vi "FTW-Request-Unknown.vi"(0 "Request":refnum<data-value>, 11 "error in":errorcluster) -> (4 "Request out":refnum<data-value>, 15 "error out":errorcluster)   [LabVIEW 2015]
uses:
  json/core/FTW-JSON-Core-Structure.ctl
  error/FTW-ERR-ThrowError.vi
  error/FTW-ERR-CallChain.vi
  error/FTW-ERR-NoErrorConstant.vi
  string/FTW-STR-ReplaceWhitespace.vi
  string/FTW-STR-Array-Delimit.vi
  error/FTW-ERR-Clear.vi
  regex/FTW-Regex-ReplaceAll.vi
panel:
  # "Inputs"
  # "Outputs"
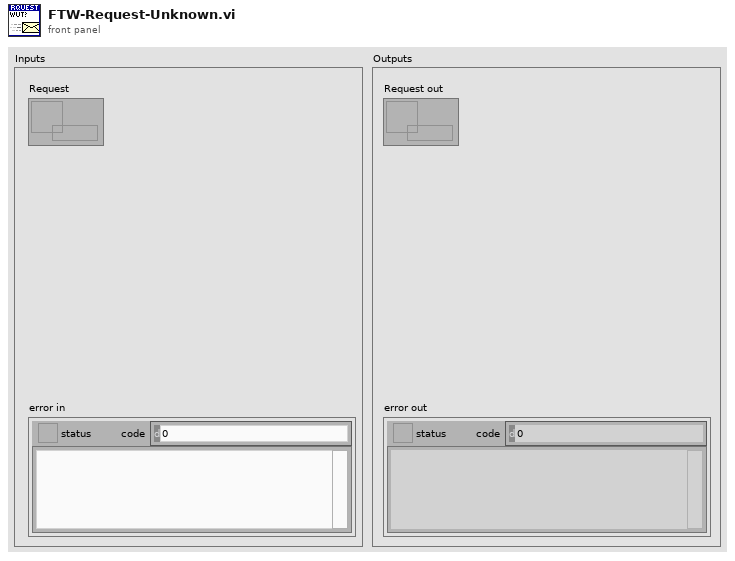
[diagram p1: front panel]
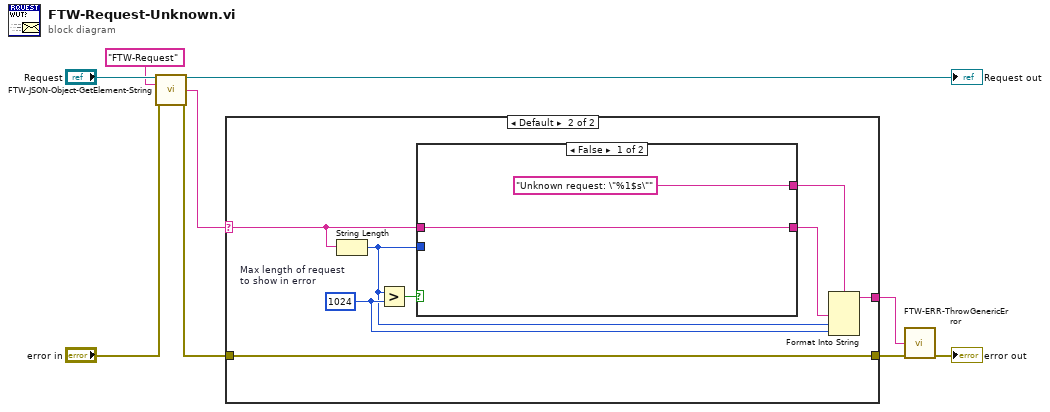
[diagram p0: block diagram]
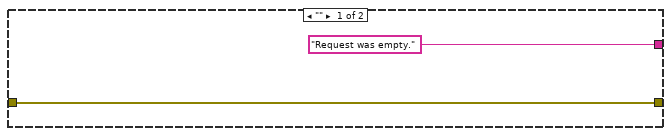
[diagram p2: hidden frame]
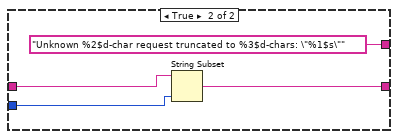
[diagram p3: hidden frame]
diagram:
  n1 = call "FTW-JSON-Object-GetElement-String.vi"("JSON Object"="Request", "Key"="FTW-Request", "error in"="error in") -> ("JSON Object out"=→"Request out":refnum<data-value>, "Value"=w3:string, "error out"=w1:errorcluster)  [unwired: 9 in, 1 out]
  n2 = case shown="Default" w3 {
    selector: w3 -> [_ w14]
    tunnel: [w10 w12] -> w9
    tunnel: w1 -> [w10 w12]
    tunnel: ["Request was empty." ("Error Message") w13] -> w7
    frame "" {
    }
    frame Default {
      w16 = 1024  # Max length of request to show in error
      n3 = String Length(string=w14) -> (length=w15:i32)
      n4 = Greater?(x=w15, y=w16) -> (0:w19:bool)
      n5 = case shown="False" w19 {
        tunnel: w14 -> [w21 w25]
        tunnel: [w21 w23] -> w18
        tunnel: ["Unknown request: \"%1$s\"" ("format string") "Unknown %2$d-char request truncated to %3$d-chars: \"%1$s\"" ("format string")] -> w17
        tunnel: w15 -> [_ w24]
        frame False {
        }
        frame True {
          n6 = String Subset(string=w25, length (rest)=w24) -> (substring=w23:string)  [unwired: 1 in]
        }
      }
      n7 = Format Into String(format string=w17, w18, w15, w16) -> (resulting string=w13:string)  [unwired: 2 in, 1 out]
    }
  }
  n8 = call "FTW-ERR-ThrowGenericError.vi"("Error Message"=w7, "error in"=w9) -> ("error out"=→"error out":errorcluster)  [unwired: 13 in]
